vi "Create Instance.vi"(8 "error in (no error)":errorcluster, 10 "Configuration":T1) -> (0 "error out":errorcluster, 3 "Power Meter out":refnum<class "Power Meter.lvclass">)   [LabVIEW 2023, in "Power Meter.lvlib" / "Power Meter.lvclass"]
uses:
  Power Meter.lvclass
  Power Meter.lvclass/Power Meter.ctl
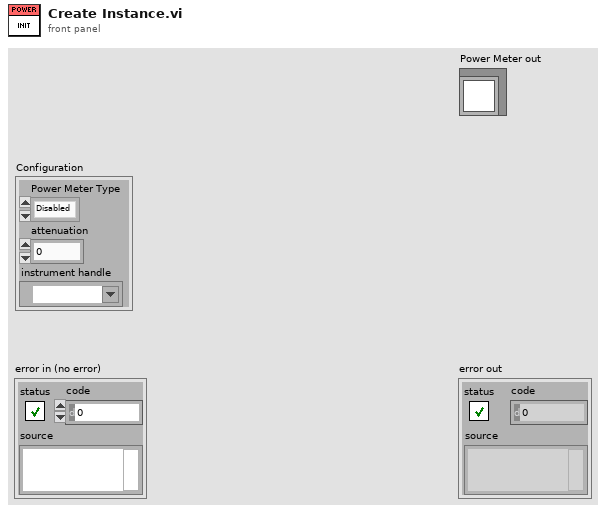
[diagram p1: front panel]
types:
  T1 = cluster{"Power Meter Type":enum16{"Disabled", "Thorlabs", "Newport", "Coherent"}, "attenuation":dbl, "instrument handle":refnum<visa-resource-name>}
  T2 = enum16{"Disabled", "Thorlabs", "Newport", "Coherent"}
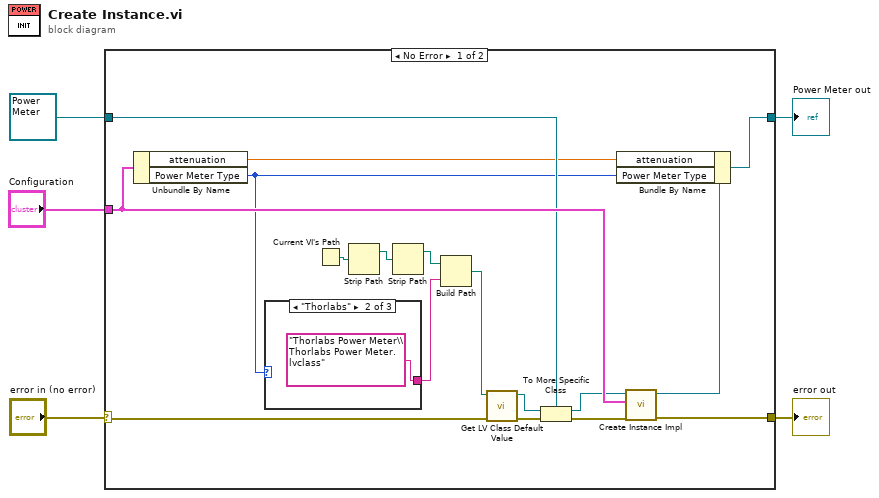
[diagram p0: block diagram]
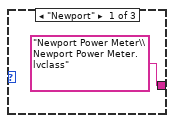
[diagram p2: hidden frame]
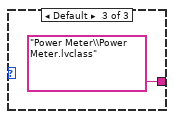
[diagram p3: hidden frame]
diagram:
  n1 = case shown="No Error" "error in (no error)" {
    selector: "error in (no error)" -> [w17 w27]
    tunnel: [w22 w27] -> w4
    tunnel: [w11 w26] -> w2
    tunnel: refnum<class "Power Meter.lvclass"> refnum ("Power Meter in") -> [w12 w26]
    tunnel: "Configuration" -> [w21 _]
    frame No Error {
      n2 = Unbundle By Name(w21) -> ("attenuation"=w9:dbl, "Power Meter Type"=w8:T2)
      n3 = case shown="\"Thorlabs\"" w8 {
        tunnel: ["Newport Power Meter\\Newport Power Meter.lvclass" "Thorlabs Power Meter\\Thorlabs Power Meter.lvclass" "Power Meter\\Power Meter.lvclass"] -> w20
        frame "Newport" {
        }
        frame "Thorlabs" {
        }
        frame Default {
        }
      }
      n4 = Current VI's Path() -> (path=w19:path)
      n5 = Strip Path(path=w19) -> (stripped path=w18:path)  [unwired: 1 out]
      n6 = Strip Path(path=w18) -> (stripped path=w7:path)  [unwired: 1 out]
      n7 = Build Path(base path=w7, name or relative path=w20) -> (appended path=w6:path)
      n8 = call <vilib>:"Get LV Class Default Value.vi"("error in (no error)"=w17, "class path"=w6) -> ("error out"=w16:errorcluster, "object"=w14:refnum<class>)  [unwired: 8 in]
      n9 = To More Specific Class(target class=w12, reference=w14, error in=w16) -> (specific class reference=w13:refnum<class "Power Meter.lvclass">, error out=w15:errorcluster)
      n10 = call-dynamic "Create Instance Impl.vi"("error in (no error)"=w15, "Configuration"=w21, "Power Meter in"=w13) -> ("error out"=w22:errorcluster, "Power Meter out"=w10:refnum<class "Power Meter.lvclass">)  [unwired: 7 in]
      n11 = Bundle By Name(cluster=w10, "attenuation"=w9, "Power Meter Type"=w8) -> (w11:refnum<class "Power Meter.lvclass">)
    }
    frame Error {
    }
  }
  "error out" <- w4
  "Power Meter out" <- w2
